vi "Get Server Internal UEs.vi"(11 "OOP Server in":refnum<class "TempController_server.lvclass">) -> (2 "Server Internal UEs":T1, 3 "OOP Server out":refnum<class "TempController_server.lvclass">)   [LabVIEW 2019, in "TempController_server.lvlib" / "TempController_server.lvclass"]
uses:
  TempController_server.lvclass
  typeDefs/Server Internal UEs.ctl
  typeDefs/Server Internal Message.ctl
  TempController_server.lvclass/TempController_server.ctl
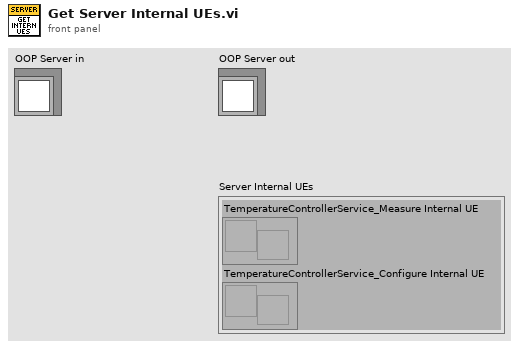
[diagram p1: front panel]
types:
  T1 = typedef "TempController_server.lvlib/TempController_server.lvclass/Server Internal UEs.ctl" = cluster{"TemperatureControllerService_Measure Internal UE":refnum<user-event>, "TemperatureControllerService_Configure Internal UE":refnum<user-event>}
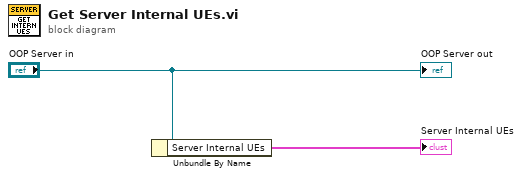
[diagram p0: block diagram]
diagram:
  n1 = Unbundle By Name("OOP Server in") -> ("Server Internal UEs"=→"Server Internal UEs":T1)
  "OOP Server out" <- "OOP Server in"
